vi "Filter Triggered.vi"(8 "error in (no error)":errorcluster, 10 "Assert Message":T1, 11 "String Filters in":refnum<class "String Filters.lvclass">) -> (0 "error out":errorcluster, 2 "Filtered":bool)   [LabVIEW 2016, in "Assert API Components.lvlib" / "String Filters.lvclass"]
uses:
  String Filters.lvclass
  Message Data.ctl
  Failure Actions.ctl
  VI References.ctl
  Base Filter.lvclass
  Assert API Components.lvlib
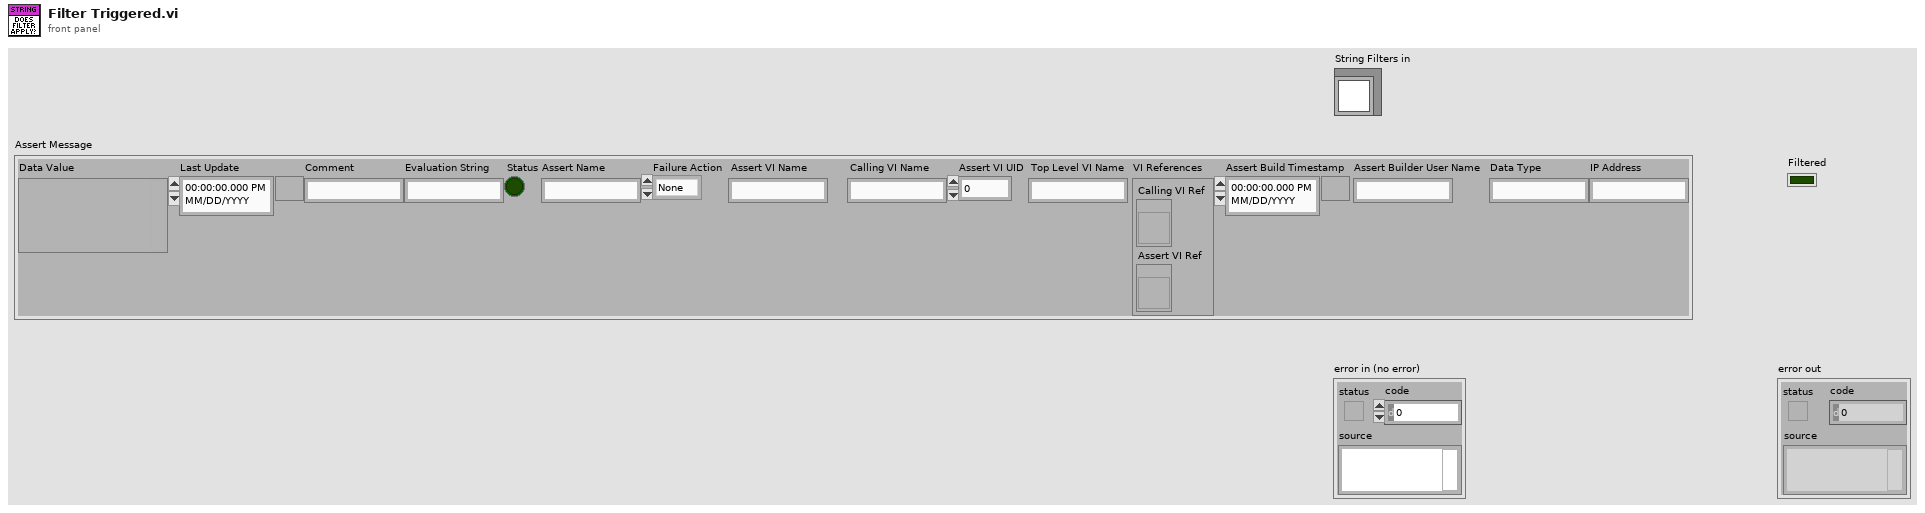
[diagram p1: front panel]
types:
  T1 = typedef "Assert API Components.lvlib/Message Data.ctl" = cluster{"Data Value":variant, "Last Update":timestamp, "Comment":string, "Evaluation String":string, "Status":bool, "Assert Name":string, "Failure Action":T2, "Assert VI Name":string, "Calling VI Name":string, "Assert VI UID":i32, "Top Level VI Name":string, "VI References":T3, "Assert Build Timestamp":timestamp, "Assert Builder User Name":string, "Data Type":string, "IP Address":string}
  T2 = typedef "Assert API Components.lvlib/Failure Actions.ctl" = enum16{"None", "Log To File", "Pause Execution", "Abort Execution"}
  T3 = typedef "Assert API Components.lvlib/VI References.ctl" = cluster{"Calling VI Ref":refnum<vi>, "Assert VI Ref":refnum<vi>}
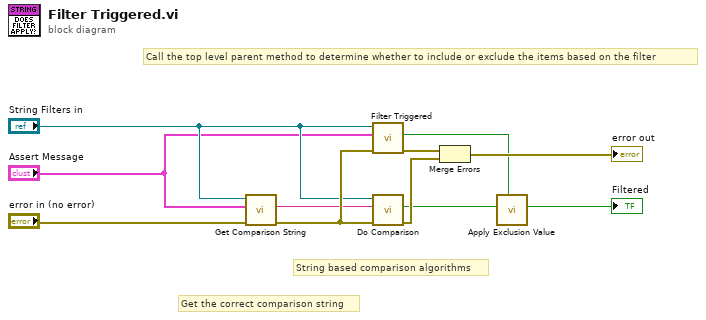
[diagram p0: block diagram]
diagram:
  # "Get the correct comparison string"
  # "String based comparison algorithms"
  # "Call the top level parent method to determine whether to include or exclude the items based on the filter"
  n1 = call-dynamic "Get Comparison String.vi"("error in (no error)"="error in (no error)", "Assert Message"="Assert Message", "String Filters in"="String Filters in") -> ("error out"=w7:errorcluster, "Comparison String"=w4:string)  [unwired: 7 in]
  n2 = call-parent "Filter Triggered.vi"("error in (no error)"=w7, "Assert Message"="Assert Message", "Base Filter in"="String Filters in") -> ("error out"=w10:errorcluster, "Filtered"=w3:bool)  [unwired: 7 in]
  n3 = call "Do Comparison.vi"("error in (no error)"=w7, "Compare String"=w4, "String Filters in"="String Filters in") -> ("error out"=w11:errorcluster, "Filtered"=w2:bool)  [unwired: 7 in]
  n4 = Merge Errors(w10, w11) -> (→"error out":errorcluster)
  n5 = call "Apply Exclusion Value.vi"("Excluded?"=w3, "Filtered value in"=w2) -> ("Final Filtered Value"=→"Filtered":bool)  [unwired: 9 in]
